vi "sub_gnss-data_check.vi"(7 "sel":T1(ring)=enum."GxGGA", 8 "error in":errorcluster, 11 "gnss str":string) -> (0 "error out":errorcluster, 1 "val":bool, 2 "LatLong":cluster{dbl, dbl} {"?" format="%.9f"; "?" format="%.9f"}, 3 "TM":cluster{dbl, dbl})   [LabVIEW 2019]
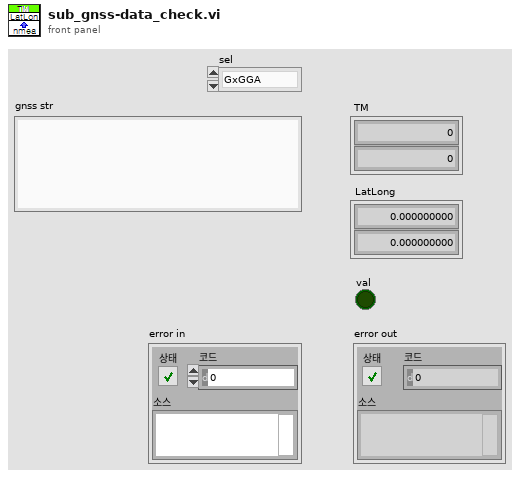
[diagram p1: front panel]
types:
  T1 = enum16{"GxDTM", "GxGBS", "GxGGA", "GxGLL", "GxGNS", "GxGRS", "GxGSA", "GxGST", "GxGSV", "GxRLM", "GxRMC", "GxTHS", "GxTXT", "GxVLW", "GxVTG", "GxZDA"}
  T2 = cluster{"lat_index":i32, "lon_index":i32, "heading index":i32}
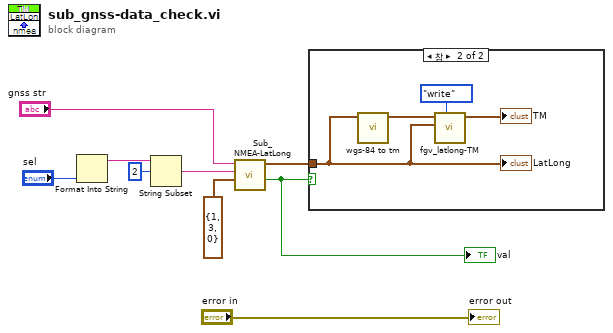
[diagram p0: block diagram]
diagram:
  n1 = Format Into String("sel") -> (resulting string=w4:string)  [unwired: 3 in, 1 out]
  n2 = String Subset(string=w4, offset (0)=2 ("오프셋(0)")) -> (substring=w2:string)  [unwired: 1 in]
  n3 = call "Sub_NMEA-LatLong.vi"("index cluster"=T2 {"lat_index"=1, "lon_index"=3, "heading index"=0}, "nmea sel"=w2, "gnss str"="gnss str") -> ("val"=w1:bool, "latlong"=w7:cluster{"Lat":dbl, "Long":dbl})  [unwired: 7 in]
  "val" <- w1
  n4 = case shown="참" w1 {
    tunnel: w7 -> [_ w10]
    frame False {
    }
    frame True {
      n5 = call "wgs-84 to tm.vi"("in_lon-lat"=w10) -> ("TM"=w12:cluster{"Y(E)":dbl, "X(N)":dbl})  [unwired: 10 in]
      n6 = call "fgv_latlong-TM.vi"("cmd"=enum16{"write", "read"}."write", "latlong"=w10, "tm"=w12) -> ("tm out"=→"TM":cluster{dbl, dbl})  [unwired: 7 in, 1 out]
      "LatLong" <- w10
    }
  }
  "error out" <- "error in"
